vi "Select Bitfile.vi"(8 "error in":errorcluster) -> (0 "error out":errorcluster, 1 "Cancelled?":bool, 2 "RIO Device Address out":string, 3 "Bitfile Path out":path)   [LabVIEW 2013, in "PWM System Explorer.lvlib"]
uses:
  PWM System Explorer.lvlib
panel:
  in  "OK":bool
  in  "Cancel":bool
  in  "Select Bitfile Path":path
  in  "RIO Device Address":string="RIO0"
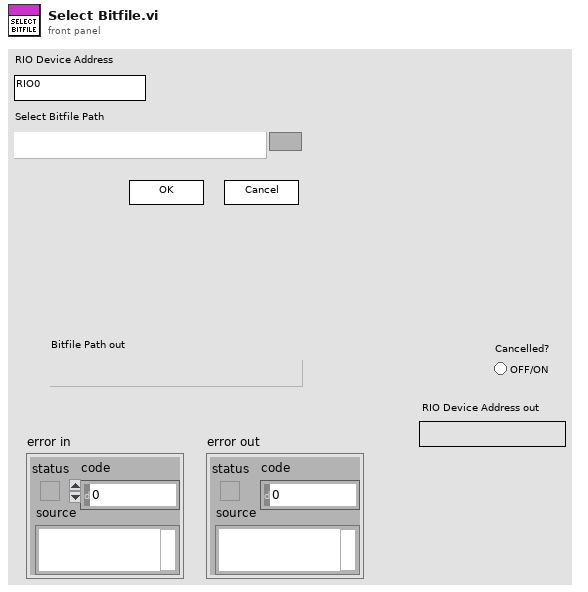
[diagram p1: front panel]
types:
  T1 = enum8{"Enabled", "Disabled", "Disabled and Grayed Out"}
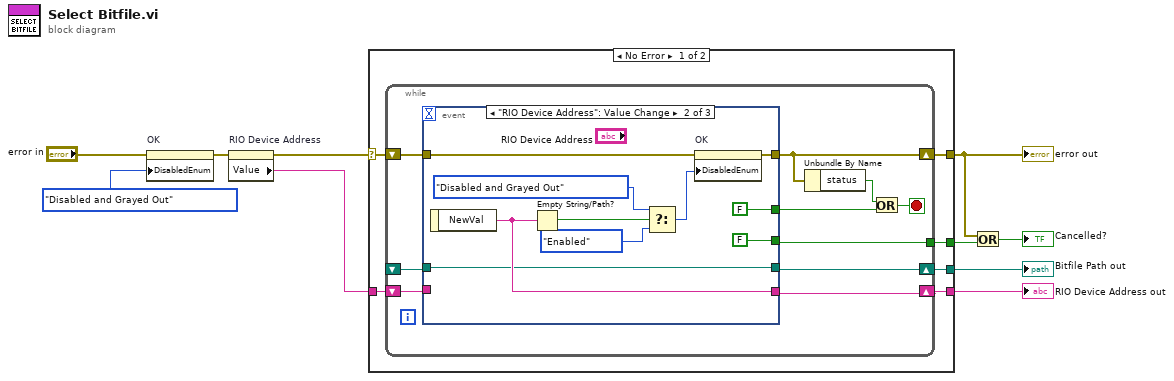
[diagram p0: block diagram]
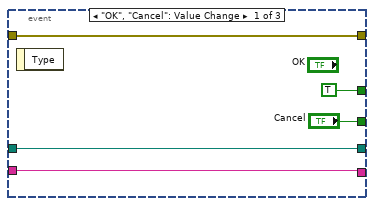
[diagram p2: hidden frame]
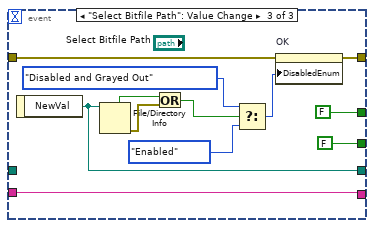
[diagram p3: hidden frame]
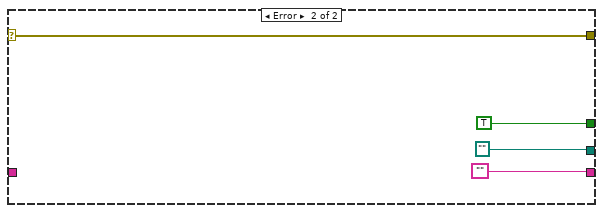
[diagram p4: hidden frame]
diagram:
  n1 = property on="OK" class="Bool"(error in="error in", "DisabledEnum"=T1."Disabled and Grayed Out" ("Disabled")) -> (error out=w3:errorcluster)  [unwired: 1 in, 1 out]
  n2 = property on="RIO Device Address" class="Str"(error in=w3) -> (error out=w2:errorcluster, "Value"=w1:string)  [unwired: 1 in, 1 out]
  n3 = case shown="No Error" w2 {
    selector: w2 -> [w16 w57]
    tunnel: [w15 w57] -> w4
    tunnel: [w14 TRUE ("Cancel")] -> w9
    tunnel: [w13 path ""] -> w6
    tunnel: [w12 ""] -> w5
    tunnel: w1 -> [w11 _]
    frame No Error {
      n4 = while {
        shift-right: [w23] -> w15
        shift-left: w16 -> [w25]
        tunnel: [w21] -> w14
        shift-right: [w20] -> w12
        shift-left: w11 -> [w19]
        shift-right: [w18] -> w13
        shift-left: _ -> [w17]
        stop <- w24 stop-if-true
        n5 = event shown="[1] \"RIO Device Address\": Value Change" {
          selector: _ -> [_ _ _]
          dyn-events: _ -> [_ _ _]
          timeout: _ -> [_ _ _]
          tunnel: [TRUE FALSE FALSE] -> w26
          tunnel: w25 -> [w29 w40 w52]
          tunnel: [w29 w41 w53] -> w23
          tunnel: ["Cancel" FALSE ("Cancel") FALSE ("Cancel")] -> w21
          tunnel: [w28 w35 w43] -> w20
          tunnel: w19 -> [w28 _ w43]
          tunnel: [w27 w33 w44] -> w18
          tunnel: w17 -> [w27 w33 _]
          event "OK", "Cancel": Value Change {
            n6 = event-data() -> ()  [unwired: 1 in, 1 out]
          }
          event "RIO Device Address": Value Change {
            n7 = event-data() -> ("NewVal"=w35:string)  [unwired: 1 in]
            n8 = Empty String/Path?(string/path=w35) -> (empty?=w37:bool)
            n9 = Select(t=T1."Disabled and Grayed Out" ("Disabled"), s=w37, f=T1."Enabled" ("Disabled")) -> (s? t:f=w36:T1)
            n10 = property on="OK" class="Bool"(error in=w40, "DisabledEnum"=w36) -> (error out=w41:errorcluster)  [unwired: 1 in, 1 out]
          }
          event "Select Bitfile Path": Value Change {
            n11 = event-data() -> ("NewVal"=w44:path)  [unwired: 1 in]
            n12 = File/Directory Info(path=w44) -> (directory=w50:bool, error out=w49:errorcluster)  [unwired: 1 in, 5 out]
            n13 = Or(x=w50, y=w49) -> (x .or. y?=w48:bool)
            n14 = Select(t=T1."Disabled and Grayed Out" ("Disabled"), s=w48, f=T1."Enabled" ("Disabled")) -> (s? t:f=w51:T1)
            n15 = property on="OK" class="Bool"(error in=w52, "DisabledEnum"=w51) -> (error out=w53:errorcluster)  [unwired: 1 in, 1 out]
          }
        }
        n16 = Unbundle By Name(w23) -> ("status"=w22:bool)
        n17 = Or(x=w22, y=w26) -> (x .or. y?=w24:bool)
      }
    }
    frame Error {
    }
  }
  "error out" <- w4
  "Bitfile Path out" <- w6
  "RIO Device Address out" <- w5
  n18 = Or(x=w4, y=w9) -> (x .or. y?=→"Cancelled?":bool)
